vi "NextMaster_v4.vi"() -> ()   [LabVIEW 2013, in "SubVIs.lvlib"]
uses:
  SubVIs.lvlib
  EvapRampNumericTriggered.ctt
  DDS/DDSUpdate.ctt
  EvapRampNumeric.ctt
  TypeDefs/Active procedure variables.ctl
  SRSRampControl_v4.ctl
  SRSDevices.ctt
  Controls.llb/Controls.lvlib
panel:
  in  "Tab Control":T1(tab)
  out "Hardware List":T4={"Master VLIW Array"=[{"Output Bits"=9470143, "Data Field"=0, "OP Code"=0, "Delay Count"=2}, {"Output Bits"=1048767, "Data Field"=0, "OP Code"=0, "Delay Count"=299999997}, {"Output Bits"=9437375, "Data Field"=0, "OP Code"=0, "Delay Count"=2}, {"Output Bits"=1048767, "Data Field"=0, "OP Code"=0, "Delay Count"=49999997}, {"Output Bits"=9437199, "Data Field"=0, "OP Code"=0, "Delay Count"=1999997}, {"Output Bits"=1048591, "Data Field"=0, "OP Code"=0, "Delay Count"=532997}, {"Output Bits"=9437231, "Data Field"=0, "OP Code"=0, "Delay Count"=599997}, {"Output Bits"=1048635, "Data Field"=0, "OP Code"=0, "Delay Count"=249997}, {"Output Bits"=9440768, "Data Field"=0, "OP Code"=0, "Delay Count"=99997}, {"Output Bits"=1052160, "Data Field"=0, "OP Code"=0, "Delay Count"=99997}, {"Output Bits"=9440768, "Data Field"=999, "OP Code"=2, "Delay Count"=2}, {"Output Bits"=1052160, "Data Field"=10, "OP Code"=3, "Delay Count"=899992}, {"Output Bits"=1052160, "Data Field"=0, "OP Code"=0, "Delay Count"=199999997}, {"Output Bits"=19968, "Data Field"=0, "OP Code"=0, "Delay Count"=532997}, {"Output Bits"=1314312, "Data Field"=0, "OP Code"=0, "Delay Count"=1249997}, {"Output Bits"=1310728, "Data Field"=0, "OP Code"=0, "Delay Count"=699997}, {"Output Bits"=9699596, "Data Field"=0, "OP Code"=0, "Delay Count"=7997}, {"Output Bits"=1310776, "Data Field"=0, "OP Code"=0, "Delay Count"=1666997}, {"Output Bits"=1310984, "Data Field"=0, "OP Code"=0, "Delay Count"=7997}, {"Output Bits"=1048605, "Data Field"=0, "OP Code"=0, "Delay Count"=2}, {"Output Bits"=1048605, "Data Field"=0, "OP Code"=0, "Delay Count"=2}, {"Output Bits"=1048605, "Data Field"=0, "OP Code"=1, "Delay Count"=97}], "Master AO Update List"=[], "Slave VLIW Array"=[{"Output Bits"=9470143, "Data Field"=0, "OP Code"=0, "Delay Count"=2}, {"Output Bits"=1048767, "Data Field"=0, "OP Code"=0, "Delay Count"=299999997}, {"Output Bits"=9437375, "Data Field"=0, "OP Code"=0, "Delay Count"=2}, {"Output Bits"=1048767, "Data Field"=0, "OP Code"=0, "Delay Count"=49999997}, {"Output Bits"=9437199, "Data Field"=0, "OP Code"=0, "Delay Count"=1999997}, {"Output Bits"=1048591, "Data Field"=0, "OP Code"=0, "Delay Count"=532997}, {"Output Bits"=9437231, "Data Field"=0, "OP Code"=0, "Delay Count"=599997}, {"Output Bits"=1048635, "Data Field"=0, "OP Code"=0, "Delay Count"=249997}, {"Output Bits"=9440768, "Data Field"=0, "OP Code"=0, "Delay Count"=99997}, {"Output Bits"=1052160, "Data Field"=0, "OP Code"=0, "Delay Count"=99997}, {"Output Bits"=9440768, "Data Field"=999, "OP Code"=2, "Delay Count"=2}, {"Output Bits"=1052160, "Data Field"=10, "OP Code"=3, "Delay Count"=899992}, {"Output Bits"=1052160, "Data Field"=0, "OP Code"=0, "Delay Count"=199999997}, {"Output Bits"=19968, "Data Field"=0, "OP Code"=0, "Delay Count"=532997}, {"Output Bits"=1314312, "Data Field"=0, "OP Code"=0, "Delay Count"=1249997}, {"Output Bits"=1310728, "Data Field"=0, "OP Code"=0, "Delay Count"=699997}, {"Output Bits"=9699596, "Data Field"=0, "OP Code"=0, "Delay Count"=7997}, {"Output Bits"=1310776, "Data Field"=0, "OP Code"=0, "Delay Count"=1666997}, {"Output Bits"=1310984, "Data Field"=0, "OP Code"=0, "Delay Count"=7997}, {"Output Bits"=1048605, "Data Field"=0, "OP Code"=0, "Delay Count"=2}, {"Output Bits"=1048605, "Data Field"=0, "OP Code"=0, "Delay Count"=2}, {"Output Bits"=1048605, "Data Field"=0, "OP Code"=1, "Delay Count"=97}], "Slave AO Update List"=[], "Master DO Update List"=[], "Slave DO Update List"=[], "Master Novatech Update List"=[], "Slave Novatech Update List"=[], "DDS Update List"=[]} {"Slave Novatech Update List"."3 phase" format="%#.5f"; "Slave Novatech Update List"."2 phase" format="%#.5f"; "Slave Novatech Update List"."3 Power [dBm]" format="%#.5f"; "Slave Novatech Update List"."3 Freq. [MHz]" format="%#_5e"; "Slave Novatech Update List"."2 Power [dBm]" format="%#.5f"; "Slave Novatech Update List"."2 Freq. [MHz]" format="%#_5e"; "Master Novatech Update List"."3 phase" format="%#.5f"; "Master Novatech Update List"."2 phase" format="%#.5f"; "Master Novatech Update List"."3 Power [dBm]" format="%#.5f"; "Master Novatech Update List"."3 Freq. [MHz]" format="%#_5e"; "Master Novatech Update List"."2 Power [dBm]" format="%#.5f"; "Master Novatech Update List"."2 Freq. [MHz]" format="%#_5e"; "Slave AO Update List"."AO Update List" format="%.2f"; "Slave VLIW Array"."Output Bits" format="%.0x"; "Master AO Update List"."AO Update List" format="%.2f"; "Master VLIW Array"."Output Bits" format="%.0x"}
  in  "Novatech Params":T5[](array[typedef]) {"Timestep [s]" format="%_6g"}
  out "Igor Inform String":string[](array[string])=["# Current Variables\n# \n# Master Staging List\n# Line\tMarker\tOption\tHalt\t0       4       8      12      16      20    AO\tDelay\t\tPoints\t0\t\t1\t\t2\t\t3\t\t4\t\t5\t\t6\t\t7\t\t8\t\t9\t\t10\t\t11\t\t12\t\t13\t\t14\t\t15\t\tComment\n00\t\tRamp\t0 0 0 0 0 0 0 0 0 0 0 0 0 0 0 0 0 0 0 0 0 0 0 0\t10e-3\t0\t0\t0\t0\t0\t\n01\t\t\t0 0 0 0 0 0 0 0 0 0 0 0 0 0 0 0 0 0 0 0 0 0 0 0\t10e-3\t0\t\t\t\t\t\n02\t\tRamp\t0 0 0 0 0 0 0 0 0 0 0 0 0 0 0 0 0 0 0 0 0 0 0 0\t10e-3\t0\tLineRamp(f, 0, 1)\t-LineRamp(f, 0, 1)\t2*LineRamp(f, 0, 1)\t-2*LineRamp(f, 0, 1)\t\n03\t\t\t0 0 0 0 0 0 0 0 0 0 0 0 0 0 0 0 0 0 0 0 0 0 0 0\t1e-3\t0\t\t\t\t\t\n04\t\tRamp\t0 0 0 0 0 0 0 0 0 0 0 0 0 0 0 0 0 0 0 0 0 0 0 0\t10e-3\t0\tSinRamp(t, 0, 1,1e3,pi/2)\t-SinRamp(t, 0, 1,1e3,pi/2)\t2*SinRamp(t, 0, 1,1e3,pi/2)\t-2*SinRamp(t, 0, 1,1e3,pi/2)\t\n05\t\tRamp\t0 0 0 0 0 0 0 0 0 0 0 0 0 0 0 0 0 0 0 0 0 0 0 0\t1e-3\t0\tLineRamp(f, 1, 2)\tLineRamp(f, 1, 2)\t2*LineRamp(f, 1, 2)\t-2*LineRamp(f, 1, 2)\t\n06\t\tRamp\t0 0 0 0 0 0 0 0 0 0 0 0 0 0 0 0 0 0 0 0 0 0 0 0\t10e-3\t0\tLineRamp(f, 2, 0)\t-LineRamp(f, 2, 0)\t2*LineRamp(f, 2, 0)\t-2*LineRamp(f, 2, 0)\t\n07\t\t\t0 0 0 0 0 0 0 0 0 0 0 0 0 0 0 0 0 0 0 0 0 0 0 0\t10e-3\t0\t\t\t\t\t\n# Slave Staging List\n# Line\tMarker\tOption\tHalt\t0       4       8      12      16      20    AO\tDelay\t\tPoints\t0\t\t1\t\t2\t\t3\t\t4\t\t5\t\t6\t\t7\t\t8\t\t9\t\t10\t\t11\t\t12\t\t13\t\t14\t\t15\t\tComment\n# SRS List\n# \n#\n# Evaporation\n# Line\tDelay [s]\tFreq [MHz] \tPower [dBm]"]
  in  "Current Variable settings Global":T6[](array[typedef])
  in  "User Procedures":string="\n-- -------------------------------------------------------------------------------------------\n-- The following functions are part of the \"standard load\" of functions and should not be messed with\n-- They are here for reference only.\n-- Please add any user functions above this comment\n-- -------------------------------------------------------------------------------------------\n\n-- Creates a linear ramp from A to B\nfunction LineRamp(f, Initial, Final)\n    return (1-f)*Initial + f*Final;\nend\n\n-- Creates an exponential ramp from A to B\nfunction ExpRamp(t, a, b, tau)\n   return (b - a*exp(tMax / tau) + (a-b)*exp(t/tau))/ ( 1 - exp(tMax / tau) );\nend\n\n-- Creates a sinewave\nfunction SinRamp(t,Offset,A,Freq, Phase)\n    return Offset + A * sin(2*pi*Freq*t + Phase)\nend\n\n-- Creates a blackman pulse\nfunction Blackman(f, Offset, A)\n    return Offset +  A*sqrt(0.5*cos(3.1415*(2*f-1))+0.08*cos(2*pi*(2*f-1))+0.42);\nend\n\n-- Creates a half-gauss ramp\nfunction HalfGaussRamp(t, a, b, Width)\n    local y;\n    y = exp(-(tMax^2)/Width^2);\n    y = (a -  b*y)/(1-y)  +  ((b-a)/(1-y))*exp(-((t-tMax)^2)/Width^2);\n    return y;\nend"
  in  "HP8673B":T7(array[cluster])
  in  "SRS Ramps":T10(array[cluster])
  out "procedure":string="23Apr09_Example"
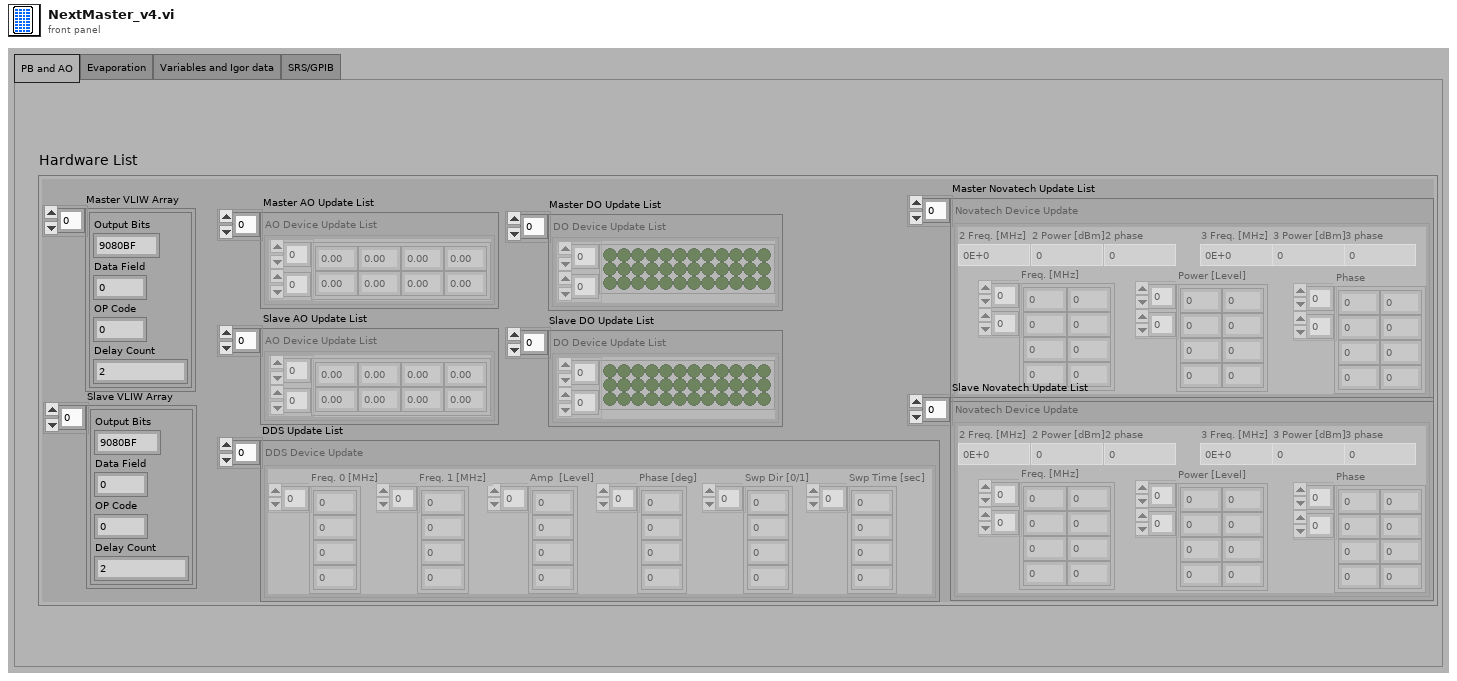
[diagram p1: front panel]
types:
  T1 = enum32{"PB and AO", "Evaporation", "Variables and Igor data", "SRS/GPIB"}
  T2 = typedef "Controls.lvlib/EvapRampNumericTriggered.ctt" = cluster{"Freq. [MHz]":dbl[][], "Power [Level]":u16[][], "Phase":u16[][], "2 Freq. [MHz]":dbl, "2 Power [dBm]":u16, "2 phase":u16, "3 Freq. [MHz]":dbl, "3 Power [dBm]":u16, "3 phase":u16}
  T3 = typedef "Controls.lvlib/DDSUpdate.ctt" = cluster{"Freq. 0 [MHz]":dbl[], "Amp  [Level]":dbl[], "Phase [deg]":dbl[], "Freq. 1 [MHz]":dbl[], "Swp Dir [0/1]":u16[], "Swp Time [sec]":dbl[]}
  T4 = cluster{"Master VLIW Array":cluster{"Output Bits":u32, "Data Field":u32, "OP Code":u8, "Delay Count":u32}[], "Master AO Update List":cluster{"AO Update List":dbl[][]}[], "Slave VLIW Array":cluster{"Output Bits":u32, "Data Field":u32, "OP Code":u8, "Delay Count":u32}[], "Slave AO Update List":cluster{"AO Update List":dbl[][]}[], "Master DO Update List":cluster{"DO Update List":bool[][]}[], "Slave DO Update List":cluster{"DO Update List":bool[][]}[], "Master Novatech Update List":T2[], "Slave Novatech Update List":T2[], "DDS Update List":T3[]}
  T5 = typedef "Controls.lvlib/EvapRampNumeric.ctt" = cluster{"2 Freq. [MHz]":dbl, "2 Power [dBm]":u16, "3 Freq. [MHz]":dbl, "3 Power [dBm]":u16, "Serial Port":refnum<visa-resource-name>, "Freq. [MHz]":dbl[][], "Power [Level]":u16[][], "Timestep [s]":dbl[]}
  T6 = typedef "Active procedure variables.ctl" = cluster{"Procedure variable":string, "Value":dbl}
  T7 = cluster{"Freq (MHz)":string, "Amp (dBm)":string, "GPIB Address":string}[]
  T8 = typedef "Controls.lvlib/SRSRampControl_v4.ctl" = cluster{"dt":string, "formula":string}
  T9 = typedef "Controls.lvlib/SRSDevices.ctt" = enum16{"1550 Vertical", "Bragg Agilent", "Bragg PTS", "Acc. Intensity"}
  T10 = cluster{"lattice ramp":T8[], "Output":cluster{"Time Values":dbl[], dbl[]}[], "SRS Selection":T9}[]
diagram:
